vi "GetParamWavePulseDelay.vi"(3 "error in (no error)":errorcluster, 4 "Selection":u8(ring) items=["Value", "Minimum", "Maximum"], 5 "ParamWave Name":string, 6 "VISA resource name":refnum<visa-resource-name>) -> (0 "error out":errorcluster, 1 "Pulse Delay [s]":dbl, 2 "VISA resource name out":refnum<visa-resource-name>)   [LabVIEW 2020, in "Active Technologies AWG3000.lvlib"]
uses:
  Active Technologies AWG3000.lvlib
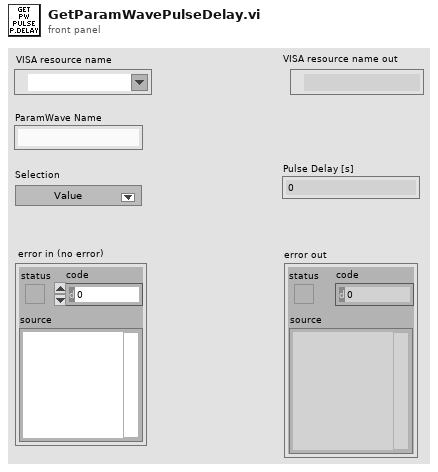
[diagram p1: front panel]
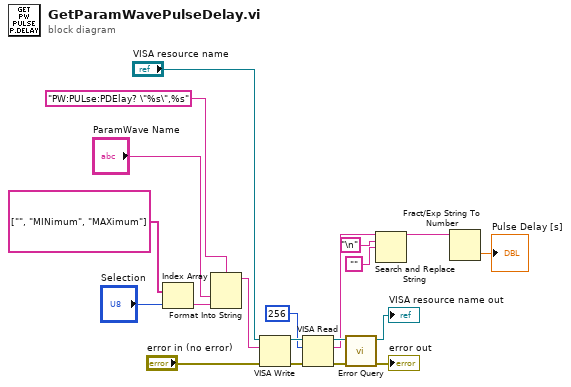
[diagram p0: block diagram]
diagram:
  n1 = Index Array(array=string[] ["", "MINimum", "MAXimum"], index="Selection") -> (element=w1:string)
  n2 = Format Into String(format string="PW:PULse:PDElay? \"%s\",%s" ("write buffer"), "ParamWave Name", w1) -> (resulting string=w3:string)  [unwired: 2 in, 1 out]
  n3 = VISA Write(VISA resource name="VISA resource name", write buffer=w3, error in (no error)="error in (no error)") -> (VISA resource name out=w17:refnum<visa-resource-name>, error out=w16:errorcluster)  [unwired: 1 out]
  n4 = VISA Read(VISA resource name=w17, byte count=u32 256, error in (no error)=w16) -> (VISA resource name out=w14:refnum<visa-resource-name>, read buffer=w4:string, error out=w13:errorcluster)  [unwired: 1 out]
  n5 = call "Error Query.vi"("error in (no error)"=w13, "VISA resource name"=w14) -> ("error out"=→"error out":errorcluster, "VISA resource name out"=→"VISA resource name out":refnum<visa-resource-name>)  [unwired: 6 in, 2 out]
  n6 = Search and Replace String(input string=w4, search string="\n", replace string="") -> (result string=w7:string)  [unwired: 5 in, 3 out]
  n7 = Fract/Exp String To Number(string=w7) -> (number=→"Pulse Delay [s]":dbl)  [unwired: 3 in, 1 out]
